vi "HFRR ADV v03 new software.vi"() -> ()   [LabVIEW 2025] (continued)
              n1799 = String Subset(string=w1941, offset (0)=45, length (rest)=9 ("length (rest)")) -> (substring=w1956:string)
              n1800 = String Subset(string=w1941, offset (0)=15, length (rest)=9 ("length (rest)")) -> (substring=w1972:string)
              n1801 = String Subset(string=w1941, offset (0)=0, length (rest)=14 ("length (rest)")) -> (substring=w1969:string)
              n1802 = String Subset(string=w1941, offset (0)=65, length (rest)=9 ("length (rest)")) -> (substring=w1959:string)
              n1803 = Fract/Exp String To Number(string=w1943) -> (number=w1940:dbl)  [unwired: 3 in, 1 out]
              n1804 = Fract/Exp String To Number(string=w1966) -> (number=w1964:dbl)  [unwired: 3 in, 1 out]
              n1805 = Fract/Exp String To Number(string=w1951) -> (number=w1949:dbl)  [unwired: 3 in, 1 out]
              n1806 = Fract/Exp String To Number(string=w1947) -> (number=w1945:dbl)  [unwired: 3 in, 1 out]
              n1807 = Fract/Exp String To Number(string=w1956) -> (number=w1954:dbl)  [unwired: 3 in, 1 out]
              n1808 = Fract/Exp String To Number(string=w1972) -> (number=w1953:dbl)  [unwired: 3 in, 1 out]
              n1809 = Fract/Exp String To Number(string=w1969) -> (number=w1965:dbl)  [unwired: 3 in, 1 out]
              n1810 = Fract/Exp String To Number(string=w1959) -> (number=w1962:dbl)  [unwired: 3 in, 1 out]
              n1811 = Add(x=w1962, y=0.0) -> (x+y=w1958:dbl)
            }
            n1812 = Delete From Array(array=w1824, index=0) -> (array with subset deleted=w1797:dbl[])  [unwired: 1 in, 1 out]
            n1813 = Delete From Array(array=w1887, index=0) -> (array with subset deleted=w1860:dbl[])  [unwired: 1 in, 1 out]
            n1814 = Delete From Array(array=w1867, index=0) -> (array with subset deleted=w1855:dbl[])  [unwired: 1 in, 1 out]
            n1815 = Delete From Array(array=w1885, index=0) -> (array with subset deleted=w1886:dbl[])  [unwired: 1 in, 1 out]
            n1816 = call-poly <vilib>:"Mean.vi"("X"=w1797) -> ("mean"=→"КОФ2 4":dbl)  [unwired: 1 out]
            n1817 = call-poly <vilib>:"Mean.vi"("X"=w1860) -> ("mean"=→"КОФ3":dbl)  [unwired: 1 out]
            n1818 = call-poly <vilib>:"Mean.vi"("X"=w1855) -> ("mean"=→"CP3":dbl)  [unwired: 1 out]
            n1819 = Delete From Array(array=w1849, index=0) -> (array with subset deleted=w1776:dbl[])  [unwired: 1 in, 1 out]
            n1820 = Delete From Array(array=w1788, index=0) -> (array with subset deleted=w1775:dbl[])  [unwired: 1 in, 1 out]
            n1821 = Delete From Array(array=w1828, index=0) -> (array with subset deleted=w1799:dbl[])  [unwired: 1 in, 1 out]
            n1822 = Delete From Array(array=w1906, index=0) -> (array with subset deleted=w1861:dbl[])  [unwired: 1 in, 1 out]
            n1823 = Delete From Array(array=w1872, index=0) -> (array with subset deleted=w1857:dbl[])  [unwired: 1 in, 1 out]
            "array w/ subset deleted" <- w1857
            n1824 = Delete From Array(array=w1903, index=0) -> (array with subset deleted=w1904:dbl[])  [unwired: 1 in, 1 out]
            n1825 = call-poly <vilib>:"Mean.vi"("X"=w1799) -> ("mean"=→"КОФ2 2":dbl)  [unwired: 1 out]
            n1826 = call-poly <vilib>:"Mean.vi"("X"=w1861) -> ("mean"=→"КОФ1":dbl)  [unwired: 1 out]
            n1827 = Bundle "Bundle"(w1776, w1775) -> (w1781:cluster{dbl[], dbl[]})  [unwired: 1 in]
            n1828 = Bundle "Bundle"(w1776, w1904) -> (w1768:cluster{dbl[], dbl[]})  [unwired: 1 in]
            n1829 = Delete From Array(array=w1783, index=0) -> (array with subset deleted=w1771:dbl[])  [unwired: 1 in, 1 out]
            n1830 = Delete From Array(array=w1784, index=0) -> (array with subset deleted=w1773:dbl[])  [unwired: 1 in, 1 out]
            n1831 = Delete From Array(array=w1894, index=0) -> (array with subset deleted=w1895:dbl[])  [unwired: 1 in, 1 out]
            n1832 = Delete From Array(array=w1782, index=0) -> (array with subset deleted=w1769:dbl[])  [unwired: 1 in, 1 out]
            n1833 = Delete From Array(array=w1876, index=0) -> (array with subset deleted=w1877:dbl[])  [unwired: 1 in, 1 out]
            n1834 = Delete From Array(array=w1901, index=0) -> (array with subset deleted=w1807:dbl[])  [unwired: 1 in, 1 out]
            n1835 = Delete From Array(array=w1847, index=0) -> (array with subset deleted=w1803:dbl[])  [unwired: 1 in, 1 out]
            n1836 = Delete From Array(array=w1883, index=0) -> (array with subset deleted=w1805:dbl[])  [unwired: 1 in, 1 out]
            n1837 = Delete From Array(array=w1843, index=0) -> (array with subset deleted=w1801:dbl[])  [unwired: 1 in, 1 out]
            n1838 = Delete From Array(array=w1892, index=0) -> (array with subset deleted=w1806:dbl[])  [unwired: 1 in, 1 out]
            n1839 = Delete From Array(array=w1845, index=0) -> (array with subset deleted=w1802:dbl[])  [unwired: 1 in, 1 out]
            n1840 = Delete From Array(array=w1826, index=0) -> (array with subset deleted=w1798:dbl[])  [unwired: 1 in, 1 out]
            n1841 = Delete From Array(array=w1870, index=0) -> (array with subset deleted=w1856:dbl[])  [unwired: 1 in, 1 out]
            n1842 = Delete From Array(array=w1897, index=0) -> (array with subset deleted=w1858:dbl[])  [unwired: 1 in, 1 out]
            n1843 = Delete From Array(array=w1874, index=0) -> (array with subset deleted=w1804:dbl[])  [unwired: 1 in, 1 out]
            n1844 = Delete From Array(array=w1841, index=0) -> (array with subset deleted=w1800:dbl[])  [unwired: 1 in, 1 out]
            n1845 = Delete From Array(array=w1822, index=0) -> (array with subset deleted=w1796:dbl[])  [unwired: 1 in, 1 out]
            n1846 = Delete From Array(array=w1866, index=0) -> (array with subset deleted=w1854:dbl[])  [unwired: 1 in, 1 out]
            n1847 = Delete From Array(array=w1879, index=0) -> (array with subset deleted=w1859:dbl[])  [unwired: 1 in, 1 out]
            n1848 = Delete From Array(array=w1889, index=0) -> (array with subset deleted=w1772:dbl[])  [unwired: 1 in, 1 out]
            n1849 = Delete From Array(array=w1899, index=0) -> (array with subset deleted=w1774:dbl[])  [unwired: 1 in, 1 out]
            n1850 = Delete From Array(array=w1881, index=0) -> (array with subset deleted=w1770:dbl[])  [unwired: 1 in, 1 out]
            n1851 = Bundle "Bundle"(w1776, w1807) -> (w1794:cluster{dbl[], dbl[]})  [unwired: 1 in]
            n1852 = Bundle "Bundle"(w1776, w1861) -> (w1795:cluster{dbl[], dbl[]})  [unwired: 1 in]
            n1853 = Bundle "Bundle"(w1807, w1803) -> (w1809:cluster{dbl[], dbl[]})  [unwired: 1 in]
            n1854 = Bundle "Bundle"(w1772, w1771) -> (w1779:cluster{dbl[], dbl[]})  [unwired: 1 in]
            n1855 = Bundle "Bundle"(w1805, w1801) -> (w1811:cluster{dbl[], dbl[]})  [unwired: 1 in]
            n1856 = Bundle "Bundle"(w1772, w1805) -> (w1915:cluster{dbl[], dbl[]})  [unwired: 1 in]
            n1857 = Bundle "Bundle"(w1772, w1801) -> (w1839:cluster{dbl[], dbl[]})  [unwired: 1 in]
            n1858 = Bundle "Bundle"(w1772, w1860) -> (w1925:cluster{dbl[], dbl[]})  [unwired: 1 in]
            n1859 = Bundle "Bundle"(w1772, w1855) -> (w1863:cluster{dbl[], dbl[]})  [unwired: 1 in]
            n1860 = Bundle "Bundle"(w1772, w1886) -> (w1910:cluster{dbl[], dbl[]})  [unwired: 1 in]
            n1861 = Bundle "Bundle"(w1806, w1802) -> (w1810:cluster{dbl[], dbl[]})  [unwired: 1 in]
            n1862 = Bundle "Bundle"(w1774, w1773) -> (w1780:cluster{dbl[], dbl[]})  [unwired: 1 in]
            n1863 = Bundle "Bundle"(w1774, w1806) -> (w1917:cluster{dbl[], dbl[]})  [unwired: 1 in]
            n1864 = Bundle "Bundle"(w1774, w1802) -> (w1840:cluster{dbl[], dbl[]})  [unwired: 1 in]
            n1865 = Bundle "Bundle"(w1774, w1856) -> (w1864:cluster{dbl[], dbl[]})  [unwired: 1 in]
            n1866 = Bundle "Bundle"(w1774, w1858) -> (w1926:cluster{dbl[], dbl[]})  [unwired: 1 in]
            n1867 = Bundle "Bundle"(w1774, w1895) -> (w1908:cluster{dbl[], dbl[]})  [unwired: 1 in]
            n1868 = Bundle "Bundle"(w1804, w1800) -> (w1812:cluster{dbl[], dbl[]})  [unwired: 1 in]
            n1869 = Bundle "Bundle"(w1770, w1769) -> (w1778:cluster{dbl[], dbl[]})  [unwired: 1 in]
            n1870 = Bundle "Bundle"(w1770, w1804) -> (w1916:cluster{dbl[], dbl[]})  [unwired: 1 in]
            n1871 = Bundle "Bundle"(w1770, w1800) -> (w1838:cluster{dbl[], dbl[]})  [unwired: 1 in]
            n1872 = Bundle "Bundle"(w1770, w1854) -> (w1862:cluster{dbl[], dbl[]})  [unwired: 1 in]
            n1873 = Bundle "Bundle"(w1770, w1859) -> (w1924:cluster{dbl[], dbl[]})  [unwired: 1 in]
            n1874 = Bundle "Bundle"(w1770, w1877) -> (w1909:cluster{dbl[], dbl[]})  [unwired: 1 in]
            n1875 = call-poly <vilib>:"Mean.vi"("X"=w1857) -> ("mean"=→"CP1":dbl)  [unwired: 1 out]
            n1876 = call-poly <vilib>:"Mean.vi"("X"=w1798) -> ("mean"=→"КОФ2 3":dbl)  [unwired: 1 out]
            n1877 = call-poly <vilib>:"Mean.vi"("X"=w1856) -> ("mean"=→"CP2":dbl)  [unwired: 1 out]
            n1878 = call-poly <vilib>:"Mean.vi"("X"=w1858) -> ("mean"=→"КОФ2":dbl)  [unwired: 1 out]
            n1879 = call-poly <vilib>:"Mean.vi"("X"=w1796) -> ("mean"=→"КОФ2 5":dbl)  [unwired: 1 out]
            n1880 = call-poly <vilib>:"Mean.vi"("X"=w1854) -> ("mean"=→"CP4":dbl)  [unwired: 1 out]
            n1881 = call-poly <vilib>:"Mean.vi"("X"=w1859) -> ("mean"=→"КОФ4":dbl)  [unwired: 1 out]
            n1882 = Bundle "Bundle"(w1776, w1803) -> (w1767:cluster{dbl[], dbl[]})  [unwired: 1 in]
            n1883 = Bundle "Bundle"(w1776, w1857) -> (w1790:cluster{dbl[], dbl[]})  [unwired: 1 in]
            n1884 = Build Array "Build Array"(w1767, w1790) -> (w1793:cluster{dbl[], dbl[]}[])
            "XY Graph 17" <- w1793
            n1885 = Build Array "Build Array"(w1781, w1780, w1779, w1778) -> (→"Frequency ( Hz )":cluster{dbl[], dbl[]}[])
            n1886 = Build Array "Build Array"(w1809, w1810, w1811, w1812) -> (→"Air Temp ( °C ) vs Humidity ( % RH )":cluster{dbl[], dbl[]}[])
            n1887 = Build Array "Build Array"(w1794, w1917, w1915, w1916) -> (→"Air Temperature  ( °C )":cluster{dbl[], dbl[]}[])
            n1888 = Build Array "Build Array"(w1767, w1840, w1839, w1838) -> (→"Humidity ( %RH )":cluster{dbl[], dbl[]}[])
            n1889 = Build Array "Build Array"(w1795, w1926, w1925, w1924) -> (→"Coefficient Of Friction":cluster{dbl[], dbl[]}[])
            n1890 = Build Array "Build Array"(w1790, w1864, w1863, w1862) -> (→"Sample Temperature ( °C )":cluster{dbl[], dbl[]}[])
            n1891 = Build Array "Build Array"(w1768, w1908, w1910, w1909) -> (→"XY Graph 13":cluster{dbl[], dbl[]}[])
            n1892 = Bundle "Bundle"(w1776, w1799) -> (w1821:cluster{dbl[], dbl[]})  [unwired: 1 in]
            n1893 = Bundle "Bundle"(w1772, w1797) -> (w1819:cluster{dbl[], dbl[]})  [unwired: 1 in]
            n1894 = Bundle "Bundle"(w1774, w1798) -> (w1820:cluster{dbl[], dbl[]})  [unwired: 1 in]
            n1895 = Bundle "Bundle"(w1770, w1796) -> (w1818:cluster{dbl[], dbl[]})  [unwired: 1 in]
            n1896 = Build Array "Build Array"(w1821, w1820, w1819, w1818) -> (→"Stroke ( mm )":cluster{dbl[], dbl[]}[])
            n1897 = local write "XY Graph 16"(w1793) -> ()
          }
          frame #2 {
          }
          frame #3 {
            n1898 = local write "Numeric 8"(0 ("Numeric 8")) -> ()
            n1899 = local write "Numeric 11"(0 ("Numeric 11")) -> ()
            n1900 = local write "Numeric 12"(0 ("Numeric 12")) -> ()
            n1901 = local write "Numeric 13"(0 ("Numeric 13")) -> ()
            n1902 = property on="OPEN" class="Bool (strict)"("Visible"=TRUE) -> ()  [unwired: 2 in, 2 out]
            n1903 = local read "String Control 2"() -> (w2093:string)
            n1904 = local read "String Control 4"() -> (w2092:string)
            n1905 = local read "String Control 6"() -> (w2091:string)
            n1906 = local read "String Control 8"() -> (w2090:string)
            n1907 = Match Pattern(string=w2093, regular expression="Samples / cycle :- ") -> (after substring=w2107:string)  [unwired: 1 in, 3 out]
            n1908 = Match Pattern(string=w2093, regular expression="Frequency :- ") -> (after substring=w2126:string)  [unwired: 1 in, 3 out]
            n1909 = Match Pattern(string=w2092, regular expression="Samples / cycle :- ") -> (after substring=w2103:string)  [unwired: 1 in, 3 out]
            n1910 = Match Pattern(string=w2092, regular expression="Frequency :- ") -> (after substring=w2121:string)  [unwired: 1 in, 3 out]
            n1911 = Match Pattern(string=w2091, regular expression="Samples / cycle :- ") -> (after substring=w2099:string)  [unwired: 1 in, 3 out]
            n1912 = Match Pattern(string=w2091, regular expression="Frequency :- ") -> (after substring=w2116:string)  [unwired: 1 in, 3 out]
            n1913 = Match Pattern(string=w2090, regular expression="Samples / cycle :- ") -> (after substring=w2095:string)  [unwired: 1 in, 3 out]
            n1914 = Match Pattern(string=w2090, regular expression="Frequency :- ") -> (after substring=w2111:string)  [unwired: 1 in, 3 out]
            n1915 = String Subset(string=w2107, length (rest)=6 ("length (rest)")) -> (substring=w2109:string)  [unwired: 1 in]
            n1916 = String Subset(string=w2126, length (rest)=9 ("length (rest)")) -> (substring=w2128:string)  [unwired: 1 in]
            n1917 = String Subset(string=w2103, length (rest)=6 ("length (rest)")) -> (substring=w2105:string)  [unwired: 1 in]
            n1918 = String Subset(string=w2121, length (rest)=9 ("length (rest)")) -> (substring=w2123:string)  [unwired: 1 in]
            n1919 = String Subset(string=w2099, length (rest)=6 ("length (rest)")) -> (substring=w2101:string)  [unwired: 1 in]
            n1920 = String Subset(string=w2116, length (rest)=9 ("length (rest)")) -> (substring=w2118:string)  [unwired: 1 in]
            n1921 = String Subset(string=w2095, length (rest)=6 ("length (rest)")) -> (substring=w2097:string)  [unwired: 1 in]
            n1922 = String Subset(string=w2111, length (rest)=9 ("length (rest)")) -> (substring=w2113:string)  [unwired: 1 in]
            n1923 = Fract/Exp String To Number(string=w2109) -> (number=w2089:dbl)  [unwired: 3 in, 1 out]
            n1924 = Fract/Exp String To Number(string=w2128) -> (number=w2129:dbl)  [unwired: 3 in, 1 out]
            n1925 = Fract/Exp String To Number(string=w2105) -> (number=w2088:dbl)  [unwired: 3 in, 1 out]
            n1926 = Fract/Exp String To Number(string=w2123) -> (number=w2124:dbl)  [unwired: 3 in, 1 out]
            n1927 = Fract/Exp String To Number(string=w2101) -> (number=w2087:dbl)  [unwired: 3 in, 1 out]
            n1928 = Fract/Exp String To Number(string=w2118) -> (number=w2119:dbl)  [unwired: 3 in, 1 out]
            n1929 = Fract/Exp String To Number(string=w2097) -> (number=w2086:dbl)  [unwired: 3 in, 1 out]
            n1930 = Fract/Exp String To Number(string=w2113) -> (number=w2114:dbl)  [unwired: 3 in, 1 out]
            n1931 = local write "sample1"(w2089) -> ()
            n1932 = local write "freq1"(w2129) -> ()
            n1933 = local write "sample2"(w2088) -> ()
            n1934 = local write "freq2"(w2124) -> ()
            n1935 = local write "sample3"(w2087) -> ()
            n1936 = local write "freq3"(w2119) -> ()
            n1937 = local write "sample4"(w2086) -> ()
            n1938 = local write "freq 4"(w2114) -> ()
          }
        }
      }
    }
    n1939 = case shown="True" w1578 {
      selector: w1578 -> [_ w1706]
      frame False {
      }
      frame True {
        n1940 = Not(x=w1706) -> (.not. x?=w1702:bool)
        n1941 = local write "service 3"(w1702) -> ()
        n1942 = local write "OPEN 6"(w1702) -> ()
        n1943 = call <vilib>:"System Exec.vi"("wait until completion? (T)"=TRUE, "command line"="C:\\LAB-IQ\\Scar View.exe") -> ("error out"=→"error out 5":errorcluster)  [unwired: 6 in, 3 out]
      }
    }
    n1944 = case shown="\"Acquire\", Default" w1589 {
      frame "Acquire", Default {
        w2602 = 0.2 ("y")
        w2607 = 1.0 ("y")
        w2608 = 0.8 ("y")
        # "Elapsed time\ncof\nstroke\nAir temp\nTemp\nHumidity"
        n1945 = disable-structure shown="Disabled" {
          frame Disabled {
            n1946 = local read "Flag"() -> (w2625:dbl)
            n1947 = local read "RUN"() -> (w2622:bool)
            n1948 = Not(x=w2622) -> (.not. x?=w2621:bool)
            n1949 = Equal?(x=w2625, y=10.0) -> (x = y?=w2623:bool)
            n1950 = And(x=w2623, y=w2621) -> (x .and. y?=w2620:bool)
            n1951 = case shown="True" w2620 {
              frame False {
              }
              frame True {
                w2626 = FALSE ("Heater Button")
                n1952 = local write "Humidity"(w2626) -> ()
                n1953 = local write "Heater Button"(w2626) -> ()
              }
            }
          }
          frame Enabled {
          }
        }
        n1954 = disable-structure shown="Disabled" {
          frame Disabled {
            n1955 = case shown="True" {
              selector: _ -> [_ _]
              frame False {
              }
              frame True {
                w2717 = TRUE ("Heater")
                n1956 = local write "Humidity"(w2717) -> ()
                n1957 = local write "Heater Button"(w2717) -> ()
                n1958 = local read "TEST STANDARD"() -> (w2720:T3)
                n1959 = local read "TEST STANDARD"() -> (w2715:T3)
                n1960 = Equal?(x=w2720, y=enum16{"ASTM D6079", "ISO 12156", "Custom"}."ISO 12156" ("Test Standard")) -> (x = y?=w2718:bool)
                n1961 = Equal?(x=w2715, y=enum16{"ASTM D6079", "ISO 12156", "Custom"}."ASTM D6079" ("Test Standard")) -> (x = y?=w2714:bool)
                n1962 = case shown="True" w2718 {
                  frame False {
                  }
                  frame True {
                    n1963 = local write "Heater"(TRUE ("Heater")) -> ()
                    n1964 = local write "airtempflg"(FALSE ("airtempflg")) -> ()
                  }
                }
                n1965 = case shown="True" w2714 {
                  frame False {
                  }
                  frame True {
                    n1966 = local write "Heater"(FALSE ("Heater")) -> ()
                    n1967 = local write "airtempflg"(TRUE ("airtempflg")) -> ()
                  }
                }
              }
            }
          }
          frame Enabled {
          }
        }
        n1968 = stacked-sequence {
          frame #0 {
            n1969 = case shown="True" "RST FF" {
              frame False {
              }
              frame True {
                w2783 = 0.0 ("X Scale.Range:Maximum")
                n1970 = property on="Frictional Force ( N )" class="WFChart (strict)"("XScale.Maximum"=600.0 ("X Scale.Range:Maximum"), "XScale.Minimum"=w2783, "YScale.Maximum"=10.0 ("Y Scale.Range:Maximum"), "YScale.Minimum"=w2783) -> ()  [unwired: 2 in, 2 out]
              }
            }
          }
          frame #1 {
            n1971 = case shown="True" "RST TEMP" {
              frame False {
              }
              frame True {
                n1972 = property on="Temperature ( Deg C )" class="WFChart (strict)"("XScale.Minimum"=0.0 ("X Scale.Range:Minimum"), "XScale.Maximum"=600.0 ("X Scale.Range:Maximum"), "YScale.Minimum"=0.0 ("Y Scale.Range:Minimum"), "YScale.Maximum"=100.0 ("Y Scale.Range:Maximum")) -> ()  [unwired: 2 in, 2 out]
              }
            }
          }
          frame #2 {
            n1973 = case shown="True" "RSTCOF" {
              frame False {
              }
              frame True {
                n1974 = property on="Coefficient of Friction" class="WFChart (strict)"("XScale.Minimum"=0.0 ("X Scale.Range:Minimum"), "XScale.Maximum"=600.0 ("X Scale.Range:Maximum"), "YScale.Maximum"=1.0 ("X Scale.Range:Minimum"), "YScale.Minimum"=0.0 ("X Scale.Range:Minimum")) -> ()  [unwired: 2 in, 2 out]
              }
            }
          }
          frame #3 {
            n1975 = case shown="True" "RSTCOF 2" {
              frame False {
              }
              frame True {
                (unwired) 100.0 ("Y Scale.Range:Maximum")
                (unwired) 0.0 ("Y Scale.Range:Minimum")
                (unwired) 600.0 ("X Scale.Range:Maximum")
                (unwired) 0.0 ("X Scale.Range:Minimum")
              }
            }
          }
          frame #4 {
            n1976 = case shown="True" "RSTCOF 3" {
              frame False {
              }
              frame True {
                n1977 = property on="Electrical Contact Resistance ( % )" class="WFChart (strict)"("XScale.Minimum"=0.0 ("X Scale.Range:Minimum"), "XScale.Maximum"=600.0 ("X Scale.Range:Maximum"), "YScale.Minimum"=0.0 ("Y Scale.Range:Minimum"), "YScale.Maximum"=100.0 ("Y Scale.Range:Maximum")) -> ()  [unwired: 2 in, 2 out]
              }
            }
          }
        }
        n1978 = disable-structure shown="Disabled" {
          frame Disabled {
            n1979 = case shown="True" {
              selector: _ -> [_ _]
              frame False {
              }
              frame True {
                n1980 = local read "zflag 2"() -> (w2684:dbl)
                n1981 = local read "yflag"() -> (w2686:dbl)
                n1982 = Equal?(x=w2686, y=2.0 ("tflag")) -> (x = y?=w2688:bool)
                n1983 = Equal?(x=w2684, y=3.0 ("tflag")) -> (x = y?=w2687:bool)
                n1984 = And(x=w2688, y=w2687) -> (x .and. y?=w2682:bool)
                n1985 = case shown="True" w2682 {
                  frame False {
                  }
                  frame True {
                    w2713 = 0.0 ("zflag")
                    n1986 = local write "zflag"(w2713) -> ()
                    n1987 = local write "zflag 2"(w2713) -> ()
                    n1988 = Delete(path (use dialog)=path "C:/LAB-IQ-NXT/WO 2449 TT.sig" ("file path (dialog if empty)")) -> (deleted path=w2712:path)  [unwired: 4 in, 2 out]
                    n1989 = Delete(path (use dialog)=path "C:/LAB-IQ-NXT/WO 2449 TRH.sig" ("file path (dialog if empty)")) -> (deleted path=w2707:path)  [unwired: 4 in, 2 out]
                    n1990 = local read "SEN.RUN HRS"() -> (w2699:dbl)
                    n1991 = local read "SENSOR TIME"() -> (w2697:dbl)
                    n1992 = call <vilib>:"compatOverwrite.vi"("overwrite (F)"=TRUE) -> ("overwrite?"=w2689:T23)
                    n1993 = call <vilib>:"compatOverwrite.vi"("overwrite (F)"=TRUE) -> ("overwrite?"=w2693:T23)
                    n1994 = local read "Total No. of Tests"() -> (w2700:dbl)
                    n1995 = Add(x=w2697, y=w2699) -> (x+y=w2698:dbl)
                    "SEN.RUN HRS" <- w2698
                    n1996 = Open/Create/Replace File(file path (use dialog)=w2712, operation (0:open)=w2689) -> (refnum out=w2690:refnum<file>, error out=w2691:errorcluster)  [unwired: 4 in, 1 out]
                    n1997 = Open/Create/Replace File(file path (use dialog)=w2707, operation (0:open)=w2693) -> (refnum out=w2694:refnum<file>, error out=w2695:errorcluster)  [unwired: 4 in, 1 out]
                    n1998 = Deny Access(4:w2691, 6:T21."deny none" ("deny mode (2)"), 7:w2690) -> (3:w2711:refnum<file>)  [unwired: 1 out]
                    n1999 = Deny Access(4:w2695, 6:T21."deny none" ("deny mode (2)"), 7:w2694) -> (3:w2703:refnum<file>)  [unwired: 1 out]
                    n2000 = Number To Decimal String(number=w2700) -> (decimal integer string=w2708:string)  [unwired: 1 in]
                    n2001 = Number To Decimal String(number=w2698) -> (decimal integer string=w2704:string)  [unwired: 1 in]
                    n2002 = Write to Binary File(file (use dialog)=w2711, data=w2708, 5:FALSE ("prepend array or string size? (T)")) -> ()  [unwired: 3 in, 3 out]
                    n2003 = Write to Binary File(file (use dialog)=w2703, data=w2704, 5:FALSE ("prepend array or string size? (T)")) -> ()  [unwired: 3 in, 3 out]
                  }
                }
              }
            }
          }
          frame Enabled {
          }
        }
        n2004 = local read "RUN"() -> (w2611:bool)
        n2005 = local read "run replace"() -> (w2615:bool)
        n2006 = local read "run replace"() -> (w2614:bool)
        n2007 = case shown="True" w2611 {
          frame False {
            n2008 = local write "run replace"(FALSE ("run replace")) -> ()
          }
          frame True {
            "run replace" <- TRUE ("run replace")
          }
        }
        n2009 = local read "RUN"() -> (w2619:bool)
        n2010 = local read "Set Temp"() -> (w2581:dbl)
        n2011 = local read "SetTemp"() -> (w2583:dbl)
        n2012 = case shown="False" w2619 {
          tunnel: [FALSE ("TEST RUNNING") TRUE ("TEST RUNNING")] -> w2618
          frame False {
            w2802 = 0.0 ("Flag")
            n2013 = local write "Elapsed time"(0.0 ("elapsedtime")) -> ()
            n2014 = local write "Time Remaining"(w2802) -> ()
            n2015 = local write "Flag"(w2802) -> ()
            n2016 = local write "Remaining Time"(w2802) -> ()
          }
          frame True {
            n2017 = local write "Flag"(10.0 ("Flag")) -> ()
          }
        }
        n2018 = case shown="False" w2615 {
          frame False {
            n2019 = local read "zflag"() -> (→"zflag 2":dbl)
            n2020 = local write "yflag"(2.0 ("tflag")) -> ()
            n2021 = local write "FLAG 4"(0.0 ("FLAG")) -> ()
          }
          frame True {
            n2022 = local write "yflag"(1.0 ("tflag")) -> ()
            n2023 = local write "zflag"(3.0 ("zflag")) -> ()
          }
        }
        n2024 = local read "acq 2"() -> (w2613:bool)
        n2025 = local read "AIR TEMP"() -> (w2576:dbl)
        n2026 = local read "Amb temp"() -> (w2580:dbl)
        n2027 = case shown="True" "Save & Continue" {
          frame False {
          }
          frame True {
            "acq 2" <- TRUE ("acq 2")
          }
        }
        n2028 = local read "Set Rh"() -> (w2582:dbl)
        n2029 = Add(x=w2583, y=w2608) -> (x+y=w2609:dbl)
        n2030 = Subtract(x=w2583, y=w2608) -> (x-y=w2610:dbl)
        n2031 = Add(x=w2581, y=w2602) -> (x+y=w2603:dbl)
        n2032 = Subtract(x=w2581, y=w2602) -> (x-y=w2604:dbl)
        n2033 = And(x=w2613, y=w2614) -> (x .and. y?=w2612:bool)
        n2034 = Greater Or Equal?(x=w2576, y=15.0) -> (x >= y?=w2577:bool)
        "powstat" <- w2577
        n2035 = local read "Humidity ( %RH )"() -> (w2579:dbl)
        n2036 = case shown="True" "Save & Continue" {
          frame False {
          }
          frame True {
            n2037 = while {
              tunnel: "0123456789abcdefghijklmnopqrstuvwxyzABCDEFGHIJKLMNOPQRSTUVWXYZ" ("string 2") -> [w2773]
              shift-right: [w2771] -> w2766
              shift-left: "" -> [w2770]
              i -> [w2780]
              stop <- w2779 stop-if-true
              n2038 = Random Number (0-1)() -> (number: 0 to 1=w2774:dbl)
              n2039 = Multiply(x=w2774, y=62.0) -> (x*y=w2776:dbl)
              n2040 = Decrement(x="Length") -> (x-1=w2769:i16)
              n2041 = To Word Integer(number=w2776) -> (16bit integer=w2777:i16)
              n2042 = String Subset(string=w2773, offset (0)=w2777, length (rest)=1 ("length (rest)")) -> (substring=w2772:string)
              n2043 = Greater Or Equal?(x=w2780, y=w2769) -> (x >= y?=w2779:bool)
              n2044 = Concatenate Strings(w2772, w2770) -> (w2771:string)
            }
            n2045 = local write "UUID"(w2766) -> ()
          }
        }
        n2046 = In Range and Coerce(upper limit=w2609, x=w2580, lower limit=w2610) -> (In Range?=w2599:bool)  [unwired: 1 out]
        n2047 = Add(x=w2582, y=w2607) -> (x+y=w2606:dbl)
        n2048 = Subtract(x=w2582, y=w2607) -> (x-y=w2605:dbl)
        n2049 = local read "TEMP"() -> (w2578:dbl)
        n2050 = case shown="True" "Save & Continue" {
          frame False {
          }
          frame True {
            n2051 = local read "Operator ID"() -> (w3072:string)
            n2052 = local read "FILE"() -> (w3078:string)
            n2053 = String Length(string=w3078) -> (length=w3076:i32)
            n2054 = String Length(string=w3072) -> (length=w3073:i32)
            n2055 = Greater?(x=w3076, y=0) -> (0:w3075:bool)
            n2056 = Greater?(x=w3073, y=0) -> (0:w3071:bool)
            n2057 = And(x=w3075, y=w3071) -> (x .and. y?=w3070:bool)
            n2058 = case shown="True" w3070 {
              frame False {
                n2059 = stacked-sequence {
                  frame #0 {
                    n2060 = One Button Dialog(message="Please Enter a File Name and Operator ID to save data !", button name ("OK")="Ok") -> ()  [unwired: 1 out]
                  }
                  frame #1 {
                    n2061 = local write "Save & Continue"(FALSE ("OK Button")) -> ()
                  }
                }
                n2062 = local write "Save & Continue"(FALSE ("OK Button")) -> ()
              }
              frame True {
                n2063 = stacked-sequence {
                  frame #0 {
                    n2064 = local read "FILE"() -> (w3084:string)
                    n2065 = call "file check.vi"("file name in"=w3084) -> ("file name out"=w3083:string)  [unwired: 9 in, 1 out]
                    n2066 = call <vilib>:"Application Directory.vi"() -> ("Application Directory"=w3094:path)
                    n2067 = Build Path(base path=w3094, name or relative path="data") -> (appended path=w3093:path)
                    n2068 = call <vilib>:"Trim Whitespace.vi"("string"=w3083) -> ("trimmed string"=w3091:string)  [unwired: 1 in]
                    n2069 = call <vilib>:"Trim Whitespace.vi"("string"=w3083) -> ("trimmed string"=w3092:string)  [unwired: 1 in]
                    n2070 = List Folder(path=w3093) -> (folder names=w3089:string[])  [unwired: 3 in, 3 out]
                    n2071 = Match Pattern(string=w3091, regular expression="_(") -> (before substring=w3088:string)  [unwired: 1 in, 3 out]
                    n2072 = for {
                      tunnel: w3089 -> [w3103] mode=indexing
                      tunnel: w3088 -> [w3101]
                      shift-right: [w3099] -> w3086
                      shift-left: bool[] [] -> [w3100]
                      n2073 = Match Pattern(string=w3103, regular expression="_(") -> (before substring=w3102:string)  [unwired: 1 in, 3 out]
                      n2074 = Equal?(x=w3102, y=w3101) -> (x = y?=w3098:bool)
                      n2075 = case shown="True" w3098 {
                        tunnel: w3098 -> [_ w3106]
                        tunnel: w3100 -> [w3105 w3108]
                        tunnel: [w3105 w3107] -> w3099
                        frame False {
                        }
                        frame True {
                          n2076 = Insert Into Array(array=w3108, new element=w3106) -> (w3107:bool[])  [unwired: 1 in]
                        }
                      }
                    }
                    n2077 = Equal?(x=w3089, y=w3088) -> (x = y?=w3097:bool[])
                    n2078 = Or Array Elements(Boolean array=w3097) -> (logical OR=w3096:bool)
                    n2079 = Array Size(array=w3086) -> (size(s)=w3085:i32)
                    n2080 = case shown="True" w3096 {
                      tunnel: w3092 -> [_ w3116]
                      tunnel: w3085 -> [_ w3109]
                      frame False {
                      }
                      frame True {
                        n2081 = Number To Decimal String(number=w3109) -> (decimal integer string=w3112:string)  [unwired: 1 in]
                        n2082 = Search/Split String(string=w3116, search string/char (-)="_(" ("regular expression")) -> (substring before match=w3114:string)  [unwired: 1 in, 2 out]
                        n2083 = Concatenate Strings(w3114, "_(" ("regular expression"), w3112, ")" ("regular expression")) -> (w3110:string)
                        n2084 = local write "FILE"(w3110) -> ()
                      }
                    }
                  }
                  frame #1 {
                    w3118 = 0.0
                    w3131 = cluster{"y":dbl, dbl, "y":dbl}[] [] ("History Data")
                    w3132 = FALSE ("Heater Button")
                    (unwired) ")!" ("string")
                    (unwired) ")" ("string")
                    w3130 = dbl[] [] ("History Data")
                    w3136 = "\r"
                    # "C:\\WinDucom\\Data\\"
                    # "C:\\LAB-IQ-NXT\\data"
                    n2085 = local write "Humidity ( %RH )"(w3118) -> ()
                    n2086 = local write "Frequency ( Hz )"(w3118) -> ()
                    n2087 = local write "Stroke 3"(w3118) -> ()
                    n2088 = local write "speedop"(0.0 ("PIDclk 2")) -> ()
                    n2089 = local write "Set Temp 2"(65.0 ("Set Temp 2")) -> ()
                    n2090 = local write "AIR TEMP"(w3118) -> ()
                    n2091 = local write "clk"(0.0 ("clk")) -> ()
                    n2092 = local write "Stroke 4"(w3118) -> ()
                    n2093 = local write "COF 2"(w3118) -> ()
                    n2094 = local write "TEMP"(w3118) -> ()
                    n2095 = local write "ecr 3"(w3118) -> ()
                    n2096 = local write "FF 3"(w3118) -> ()
                    n2097 = local write "FF 2"(w3118) -> ()
                    n2098 = property on="Humidity ( %RH )" class="WFChart (strict)"("History Data"=w3130) -> ()  [unwired: 2 in, 2 out]
                    n2099 = property on="Coefficient of Friction" class="WFChart (strict)"("History Data"=w3130) -> ()  [unwired: 2 in, 2 out]
                    n2100 = property on="Coefficient of Friction" class="WFChart (strict)"("History Data"=w3130) -> ()  [unwired: 2 in, 2 out]
                    n2101 = property on="Frictional Force ( N )" class="WFChart (strict)"("History Data"=w3130) -> ()  [unwired: 2 in, 2 out]
                    n2102 = property on="Electrical Contact Resistance ( % )" class="WFChart (strict)"("History Data"=w3130) -> ()  [unwired: 2 in, 2 out]
                    n2103 = property on="Electrical Contact Resistance ( % )" class="WFChart (strict)"("History Data"=w3130) -> ()  [unwired: 2 in, 2 out]
                    n2104 = property on="Temperature ( Deg C )" class="WFChart (strict)"("History Data"=w3130) -> ()  [unwired: 2 in, 2 out]
                    n2105 = property on="Frictional Force ( N )" class="WFChart (strict)"("History Data"=w3130) -> ()  [unwired: 2 in, 2 out]
                    n2106 = property on="Coefficient of Friction" class="WFChart (strict)"("History Data"=w3130) -> ()  [unwired: 2 in, 2 out]
                    n2107 = property on="Frictional Force ( N )" class="WFChart (strict)"("History Data"=w3130) -> ()  [unwired: 2 in, 2 out]
                    n2108 = property on="Electrical Contact Resistance ( % )" class="WFChart (strict)"("History Data"=w3130) -> ()  [unwired: 2 in, 2 out]
                    n2109 = property on="Temperature ( Deg C )" class="WFChart (strict)"("History Data"=w3130) -> ()  [unwired: 2 in, 2 out]
                    n2110 = property on="Humidity ( %RH )" class="WFChart (strict)"("History Data"=w3130) -> ()  [unwired: 2 in, 2 out]
                    n2111 = property on="Stroke ( mm )" class="WFChart (strict)"("History Data"=w3131) -> ()  [unwired: 2 in, 2 out]
                    n2112 = property on="Stroke ( mm )" class="WFChart (strict)"("History Data"=w3131) -> ()  [unwired: 2 in, 2 out]
                    n2113 = local write "Humidity"(w3132) -> ()
                    n2114 = local write "Heater Button"(w3132) -> ()
                    n2115 = local read "FILE"() -> (w3126:string)
                    n2116 = disable-structure shown="Enabled" {
                      disable-tunnel: [w3171 _] -> w3117
                      frame Enabled {
                        n2117 = local read "NORMAL LOAD"() -> (w3171:dbl)
                      }
                      frame Disabled {
                      }
                    }
                    n2118 = call "file check.vi"("file name in"=w3126) -> ("error out"=w3129:errorcluster, "file name out"=w3123:string)  [unwired: 9 in]
                    n2119 = call "FILE PATH CREATION.vi"("error in"=w3129, "FILE NAME :"=w3123) -> ("FILE OUT"=w3122:path)  [unwired: 8 in, 1 out]
                    n2120 = Concatenate Strings(w3123, ".dgf" ("Substring")) -> (w3128:string)
                    n2121 = Concatenate Strings(w3123, ".duf" ("Substring")) -> (w3124:string)
                    n2122 = Multiply(x=w3117, y=1.0) -> (x*y=w3150:dbl)
                    n2123 = Build Path(base path=w3122, name or relative path=w3128) -> (appended path=w3121:path)
                    n2124 = Build Path(base path=w3122, name or relative path=w3124) -> (appended path=w3120:path)
                    n2125 = Number To Fractional String(number=w3150, width (-)=i16 5, precision (6)=i16 2) -> (F-format string=w3158:string)  [unwired: 1 in]
                    n2126 = local read "Fuel Discription :"() -> (w3146:string)
                    n2127 = local read "Batch Ref Num :"() -> (w3134:string)
                    n2128 = Get Date/Time String(date format (0)=enum16{"short", "long", "abbreviated"}."short") -> (date string=w3169:string, time string=w3166:string)  [unwired: 2 in]
                    n2129 = local read "Remarks :"() -> (w3145:string)
                    n2130 = Concatenate Strings("Load :- " ("Substring"), w3158, " grams ," ("Substring")) -> (w3157:string)
                    n2131 = local read "String 41"() -> (w3137:string)
                    n2132 = Concatenate Strings(w3146) -> (w3147:string)
                    n2133 = Concatenate Strings(w3134) -> (w3133:string)
                    n2134 = Concatenate Strings("tested by") -> (w3141:string)
                    n2135 = Concatenate Strings("(" ("Substring"), w3169, ")" ("Substring"), w3166) -> (w3139:string)
                    "concatenated string" <- w3139
                    n2136 = Concatenate Strings(w3145, "," ("string")) -> (w3144:string)
                    n2137 = Concatenate Strings("  TIME;      COF;       STROKE;     AIR TEMP;  TEMP;  HUMIDITY;  ECR; PID-OUT; FREQUENCY" ("Substring"), "\r") -> (w3153:string)
                    n2138 = Concatenate Strings(w3137, w3136, "Fuel Discription :-" ("Substring"), w3147, w3136, w3157, w3136, "Batch Ref Num :-" ("Substring"), w3133, w3136, " Remarks :- " ("Substring"), w3144, w3136, " Date :- " ("Substring"), w3139, w3136, "Tested By :-" ("Substring"), w3141) -> (w3151:string)
                    "REMARKS" <- w3151
                    n2139 = call <vilib>:"Write Characters To File.vi"("append to file? (new file:F)"=FALSE, "character string"=w3153, "file path (dialog if empty)"=w3121) -> ()  [unwired: 2 in, 1 out]
                    n2140 = call <vilib>:"Write Characters To File.vi"("append to file? (new file:F)"=FALSE, "character string"=w3151, "file path (dialog if empty)"=w3120) -> ()  [unwired: 2 in, 1 out]
                  }
                  frame #2 {
                    n2141 = local write "Cycles elapsed"(0 ("Cycles elapsed")) -> ()
                    n2142 = local write "cyclecount"(0 ("cyclecount")) -> ()
                    n2143 = local write "Save & Continue"(FALSE ("OK")) -> ()
                    n2144 = local write "autostrtflg"(TRUE ("autostrtflg")) -> ()
                    n2145 = local write "Save"(FALSE ("Save")) -> ()
                    n2146 = Get Date/Time In Seconds() -> (seconds since 1Jan1904=w3176:timestamp)
                    n2147 = To Double Precision Float(number=w3176) -> (double precision float=w3175:dbl)
                    n2148 = local write "acq timer"(w3175) -> ()
                    n2149 = One Button Dialog(message="Please ensure sample is mounted properly and machine is ready in all aspects for testing !", button name ("OK")="Ok") -> ()  [unwired: 1 out]
                  }
                  frame #3 {
                    n2150 = stacked-sequence {
                      frame #0 {
                        n2151 = local write "Main Dashboard Buttons"(T1."Dashboard" ("Main Dashboard Buttons")) -> ()
                        n2152 = local write "Main Tab"(T2."Acquire" ("Main Tab")) -> ()
                      }
                      frame #1 {
                        n2153 = local write "EVENT LOG"("" ("EVENT LOG")) -> ()
                      }
                      frame #2 {
                        n2154 = Wait (ms)(milliseconds to wait=u32 50) -> ()  [unwired: 1 out]
                      }
                      frame #3 {
                        n2155 = disable-structure shown="Disabled" {
                          frame Disabled {
                            n2156 = local read "EVENT LOG"() -> (w3188:string)
                            n2157 = call "Event Log.vi"("Content"="Test Details", "EVENT LOG"=w3188) -> ("EVENT LOG"=w3187:string)  [unwired: 8 in, 1 out]
                            n2158 = local write "EVENT LOG"(w3187) -> ()
                          }
                          frame Enabled {
                          }
                        }
                      }
                      frame #4 {
                        n2159 = Wait (ms)(milliseconds to wait=u32 50) -> ()  [unwired: 1 out]
                      }
                      frame #5 {
                        n2160 = local read "FILE"() -> (w3190:string)
                        n2161 = Concatenate Strings("File Name :" ("Content"), w3190) -> (w3191:string)
                        n2162 = local read "EVENT LOG"() -> (w3194:string)
                        n2163 = call "Event Log.vi"("Content"=w3191, "EVENT LOG"=w3194) -> ("EVENT LOG"=w3193:string)  [unwired: 8 in, 1 out]
                        n2164 = local write "EVENT LOG"(w3193) -> ()
                      }
                      frame #6 {
                        n2165 = Wait (ms)(milliseconds to wait=u32 50) -> ()  [unwired: 1 out]
                      }
                      frame #7 {
                        n2166 = local read "Batch Ref Num :"() -> (w3196:string)
                        n2167 = Concatenate Strings("Batch Ref No :" ("Content"), w3196) -> (w3197:string)
                        n2168 = local read "EVENT LOG"() -> (w3200:string)
                        n2169 = call "Event Log.vi"("Content"=w3197, "EVENT LOG"=w3200) -> ("EVENT LOG"=w3199:string)  [unwired: 8 in, 1 out]
                        n2170 = local write "EVENT LOG"(w3199) -> ()
                      }
                      frame #8 {
                        n2171 = Wait (ms)(milliseconds to wait=u32 50) -> ()  [unwired: 1 out]
                      }
                      frame #9 {
                        n2172 = local read "tested by"() -> (w3202:string)
                        n2173 = Concatenate Strings("Tested By :" ("Content"), w3202) -> (w3203:string)
                        n2174 = local read "EVENT LOG"() -> (w3206:string)
                        n2175 = call "Event Log.vi"("Content"=w3203, "EVENT LOG"=w3206) -> ("EVENT LOG"=w3205:string)  [unwired: 8 in, 1 out]
                        n2176 = local write "EVENT LOG"(w3205) -> ()
                      }
                      frame #10 {
                        n2177 = Wait (ms)(milliseconds to wait=u32 50) -> ()  [unwired: 1 out]
                      }
                      frame #11 {
                        n2178 = local read "TEST STANDARD"() -> (w3209:T3)
                        n2179 = case shown="\"ASTM D6079\", Default" w3209 {
                          tunnel: ["ASTM D6079" "ISO 12156" "CEC F-096-A-06" "Custom"] -> w3208
                          frame "ASTM D6079", Default {
                          }
                          frame "ISO 12156" {
                          }
                          frame "CEC F-096-A-06" {
                          }
                          frame "Custom" {
                          }
                        }
                        n2180 = Concatenate Strings("Test Standard :" ("Content"), w3208) -> (w3210:string)
                        n2181 = local read "EVENT LOG"() -> (w3213:string)
                        n2182 = call "Event Log.vi"("Content"=w3210, "EVENT LOG"=w3213) -> ("EVENT LOG"=w3212:string)  [unwired: 8 in, 1 out]
                        n2183 = local write "EVENT LOG"(w3212) -> ()
                      }
                      frame #12 {
                        n2184 = Wait (ms)(milliseconds to wait=u32 50) -> ()  [unwired: 1 out]
                      }
                      frame #13 {
                        n2185 = local read "Fuel Discription :"() -> (w3219:string)
                        n2186 = Concatenate Strings("Fuel Description :" ("Content"), w3219) -> (w3220:string)
                        n2187 = local read "EVENT LOG"() -> (w3223:string)
                        n2188 = call "Event Log.vi"("Content"=w3220, "EVENT LOG"=w3223) -> ("EVENT LOG"=w3222:string)  [unwired: 8 in, 1 out]
                        n2189 = local write "EVENT LOG"(w3222) -> ()
                      }
                      frame #14 {
                        n2190 = Wait (ms)(milliseconds to wait=u32 50) -> ()  [unwired: 1 out]
                      }
                      frame #15 {
                        n2191 = local read "Remarks :"() -> (w3225:string)
                        n2192 = Concatenate Strings("Remarks :" ("Content"), w3225) -> (w3226:string)
                        n2193 = local read "EVENT LOG"() -> (w3229:string)
                        n2194 = call "Event Log.vi"("Content"=w3226, "EVENT LOG"=w3229) -> ("EVENT LOG"=w3228:string)  [unwired: 8 in, 1 out]
                        n2195 = local write "EVENT LOG"(w3228) -> ()
                      }
                      frame #16 {
                        n2196 = Wait (ms)(milliseconds to wait=u32 50) -> ()  [unwired: 1 out]
                      }
                      frame #17 {
                        n2197 = local read "Operator ID"() -> (w3231:string)
                        n2198 = Concatenate Strings("Operator ID :" ("Content"), w3231) -> (w3233:string)
                        n2199 = local read "EVENT LOG"() -> (w3235:string)
                        n2200 = call "Event Log.vi"("Content"=w3233, "EVENT LOG"=w3235) -> ("EVENT LOG"=w3234:string)  [unwired: 8 in, 1 out]
                        n2201 = local write "EVENT LOG"(w3234) -> ()
                      }
                      frame #18 {
                        n2202 = Wait (ms)(milliseconds to wait=u32 50) -> ()  [unwired: 1 out]
                      }
                      frame #19 {
                        n2203 = disable-structure shown="Disabled" {
                          frame Disabled {
                            n2204 = local read "EVENT LOG"() -> (w3239:string)
                            n2205 = call "Event Log.vi"("Content"="Test Parameter", "EVENT LOG"=w3239) -> ("EVENT LOG"=w3238:string)  [unwired: 8 in, 1 out]
                            n2206 = local write "EVENT LOG"(w3238) -> ()
                          }
                          frame Enabled {
                          }
                        }
                      }
                      frame #20 {
                        n2207 = Wait (ms)(milliseconds to wait=u32 50) -> ()  [unwired: 1 out]
                      }
                      frame #21 {
                        n2208 = local read "Set Hz"() -> (w3243:dbl)
                        n2209 = Number To Fractional String(number=w3243, precision (6)=i16 2) -> (F-format string=w3242:string)  [unwired: 2 in]
                        n2210 = Concatenate Strings("Set Frequency [Hz] :" ("Content"), w3242) -> (w3245:string)
                        n2211 = local read "EVENT LOG"() -> (w3247:string)
                        n2212 = call "Event Log.vi"("Content"=w3245, "EVENT LOG"=w3247) -> ("EVENT LOG"=w3246:string)  [unwired: 8 in, 1 out]
                        n2213 = local write "EVENT LOG"(w3246) -> ()
                      }
                      frame #22 {
                        n2214 = Wait (ms)(milliseconds to wait=u32 50) -> ()  [unwired: 1 out]
                      }
                      frame #23 {
                        n2215 = local read "NORMAL LOAD"() -> (w3250:dbl)
                        n2216 = Number To Fractional String(number=w3250, precision (6)=i16 2) -> (F-format string=w3251:string)  [unwired: 2 in]
                        n2217 = Concatenate Strings("Applied Load [grams] :" ("Content"), w3251) -> (w3253:string)
                        n2218 = local read "EVENT LOG"() -> (w3255:string)
                        n2219 = call "Event Log.vi"("Content"=w3253, "EVENT LOG"=w3255) -> ("EVENT LOG"=w3254:string)  [unwired: 8 in, 1 out]
                        n2220 = local write "EVENT LOG"(w3254) -> ()
                      }
                      frame #24 {
                        n2221 = Wait (ms)(milliseconds to wait=u32 50) -> ()  [unwired: 1 out]
                      }
                      frame #25 {
                        n2222 = local read "Set Strk"() -> (w3258:dbl)
                        n2223 = Number To Fractional String(number=w3258, precision (6)=i16 2) -> (F-format string=w3259:string)  [unwired: 2 in]
                        n2224 = Concatenate Strings("Set Stroke [mm] :" ("Content"), w3259) -> (w3261:string)
                        n2225 = local read "EVENT LOG"() -> (w3263:string)
                        n2226 = call "Event Log.vi"("Content"=w3261, "EVENT LOG"=w3263) -> ("EVENT LOG"=w3262:string)  [unwired: 8 in, 1 out]
                        n2227 = local write "EVENT LOG"(w3262) -> ()
                      }
                      frame #26 {
                        n2228 = Wait (ms)(milliseconds to wait=u32 50) -> ()  [unwired: 1 out]
                      }
                      frame #27 {
                        n2229 = local read "Set Temp"() -> (w3266:dbl)
                        n2230 = Number To Fractional String(number=w3266, precision (6)=i16 2) -> (F-format string=w3267:string)  [unwired: 2 in]
                        n2231 = Concatenate Strings("Set Temperature [deg C] :" ("Content"), w3267) -> (w3269:string)
                        n2232 = local read "EVENT LOG"() -> (w3271:string)
                        n2233 = call "Event Log.vi"("Content"=w3269, "EVENT LOG"=w3271) -> ("EVENT LOG"=w3270:string)  [unwired: 8 in, 1 out]
                        n2234 = local write "EVENT LOG"(w3270) -> ()
                      }
                      frame #28 {
                        n2235 = Wait (ms)(milliseconds to wait=u32 50) -> ()  [unwired: 1 out]
                      }
                      frame #29 {
                        n2236 = local read "Set Rh"() -> (w3274:dbl)
                        n2237 = Number To Fractional String(number=w3274, precision (6)=i16 2) -> (F-format string=w3275:string)  [unwired: 2 in]
                        n2238 = Concatenate Strings("Set Humidity [%RH] :" ("Content"), w3275) -> (w3277:string)
                        n2239 = local read "EVENT LOG"() -> (w3279:string)
                        n2240 = call "Event Log.vi"("Content"=w3277, "EVENT LOG"=w3279) -> ("EVENT LOG"=w3278:string)  [unwired: 8 in, 1 out]
                        n2241 = local write "EVENT LOG"(w3278) -> ()
                      }
                      frame #30 {
                        n2242 = Wait (ms)(milliseconds to wait=u32 50) -> ()  [unwired: 1 out]
                      }
                      frame #31 {
                        n2243 = local read "test time"() -> (w3282:dbl)
                        n2244 = Number To Fractional String(number=w3282, precision (6)=i16 1) -> (F-format string=w3283:string)  [unwired: 2 in]
                        n2245 = Concatenate Strings("Test Duration [mins] :" ("Content"), w3283) -> (w3285:string)
                        n2246 = local read "EVENT LOG"() -> (w3287:string)
                        n2247 = call "Event Log.vi"("Content"=w3285, "EVENT LOG"=w3287) -> ("EVENT LOG"=w3286:string)  [unwired: 8 in, 1 out]
                        n2248 = local write "EVENT LOG"(w3286) -> ()
                      }
                      frame #32 {
                        w3288 = dbl[] [] ("History Data")
                        w3289 = cluster{"y":dbl, dbl, "y":dbl}[] [] ("History Data")
                        w3290 = FALSE ("Visible")
                        n2249 = property on="Stroke ( mm )" class="WFChart (strict)"("History Data"=w3289) -> ()  [unwired: 2 in, 2 out]
                        n2250 = property on="Humidity ( %RH )" class="WFChart (strict)"("History Data"=w3288) -> ()  [unwired: 2 in, 2 out]
                        n2251 = property on="Temperature ( Deg C )" class="WFChart (strict)"("History Data"=w3288) -> ()  [unwired: 2 in, 2 out]
                        n2252 = property on="Electrical Contact Resistance ( % )" class="WFChart (strict)"("History Data"=w3288) -> ()  [unwired: 2 in, 2 out]
                        n2253 = property on="Coefficient of Friction" class="WFChart (strict)"("History Data"=w3288) -> ()  [unwired: 2 in, 2 out]
                        n2254 = property on="Frictional Force ( N )" class="WFChart (strict)"("History Data"=w3288) -> ()  [unwired: 2 in, 2 out]
                        n2255 = property on="Coefficient of Friction" class="WFChart (strict)"("History Data"=w3288) -> ()  [unwired: 2 in, 2 out]
                        n2256 = property on="Frictional Force ( N )" class="WFChart (strict)"("History Data"=w3288) -> ()  [unwired: 2 in, 2 out]
                        n2257 = property on="Electrical Contact Resistance ( % )" class="WFChart (strict)"("History Data"=w3288) -> ()  [unwired: 2 in, 2 out]
                        n2258 = property on="Humidity ( %RH )" class="WFChart (strict)"("History Data"=w3288) -> ()  [unwired: 2 in, 2 out]
                        n2259 = property on="Stroke ( mm )" class="WFChart (strict)"("History Data"=w3289) -> ()  [unwired: 2 in, 2 out]
                        n2260 = property on="Temperature ( Deg C )" class="WFChart (strict)"("History Data"=w3288) -> ()  [unwired: 2 in, 2 out]
                        n2261 = property on="Service Password Log" class="Str"("Visible"=w3290) -> ()  [unwired: 2 in, 2 out]
                        n2262 = property on="Password 3" class="Clust (strict)"("Visible"=w3290) -> ()  [unwired: 2 in, 2 out]
                      }
                    }
                    "TEST FILE NAM,E SAVED" <- TRUE ("TEST FILE NAM,E SAVED")
                  }
                }
              }
            }
          }
        }
        n2263 = case shown="True" w2612 {
          frame False {
            n2264 = local write "tfalg"(0.0 ("tfalg")) -> ()
          }
          frame True {
            n2265 = local read "tfalg"() -> (w2757:dbl)
            n2266 = Equal?(x=w2757, y=0.0) -> (x = y?=w2758:bool)
            n2267 = case shown="True" w2758 {
              frame False {
              }
              frame True {
                n2268 = local read "Total No. of Tests"() -> (w2761:dbl)
                n2269 = local write "tfalg"(1.0 ("tfalg")) -> ()
                n2270 = local write "acq 2"(FALSE ("acq 2")) -> ()
                n2271 = Wait (ms)(milliseconds to wait=u32 200) -> ()  [unwired: 1 out]
                n2272 = Increment(x=w2761) -> (x+1=w2760:dbl)
                n2273 = local write "Total No. of Tests"(w2760) -> ()
              }
            }
          }
        }
        n2274 = local write "Test \nStatus"(w2618) -> ()
        n2275 = local write "Save"(w2618) -> ()
        n2276 = local read "Main Tab"() -> (w2575:T2)
        n2277 = case shown="True" w2599 {
          tunnel: [FALSE ("RUN") TRUE ("RUN")] -> w2598
          tunnel: [_ 1] -> w2591
          frame False {
          }
          frame True {
          }
        }
        n2278 = In Range and Coerce(upper limit=w2606, x=w2579, lower limit=w2605) -> (In Range?=w2597:bool)  [unwired: 1 out]
        n2279 = In Range and Coerce(upper limit=w2603, x=w2578, lower limit=w2604) -> (In Range?=w2595:bool)  [unwired: 1 out]
        n2280 = case shown="True" w2611 {
          frame False {
            n2281 = local read "Rt 3"() -> (w2739:bool)
            n2282 = case shown="True" w2739 {
              frame False {
